vi "Create OPC UA Name.vi"(7 "Parent Type":T1, 11 "SV":string) -> (3 "Path":string, 4 "Folder":string, 5 "Name":string)   [LabVIEW 2016]
doc: "Generates an OPC UA name and position for the shared variable."
uses:
  Controls/Node Type.ctl
  <vilib>/OPCUA/NI OPC UA Utility.lvlib
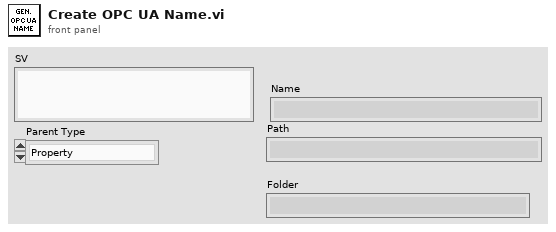
[diagram p1: front panel]
types:
  T1 = typedef "Node Type.ctl" = enum16{"Property", "Item", "Folder"}
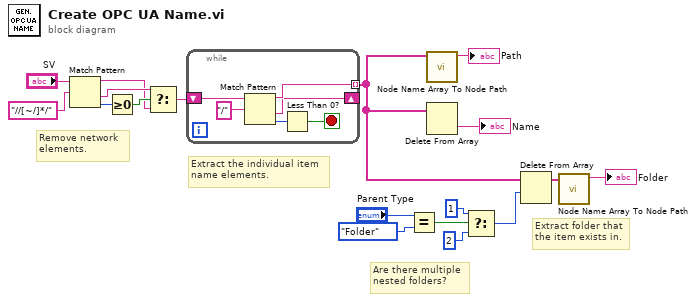
[diagram p0: block diagram]
diagram:
  # "Remove network\nelements."
  # "Extract the individual item\nname elements."
  # "Extract folder that\nthe item exists in."
  # "Are there multiple\nnested folders?"
  n1 = Match Pattern(string="SV", regular expression="//[~/]*/") -> (before substring=w14:string, after substring=w15:string, offset past match=w17:i32)  [unwired: 1 in, 1 out]
  n2 = Greater Or Equal To 0?(x=w17) -> (x >= 0?=w16:bool)
  n3 = Select(t=w15, s=w16, f=w14) -> (s? t:f=w10:string)
  n4 = while {
    shift-right: [w19] -> _
    shift-left: w10 -> [w24]
    tunnel: [w20] -> w8 mode=indexing
    stop <- w21 stop-if-true
    n5 = Match Pattern(string=w24, regular expression="/" ("regular expression (\"\")")) -> (before substring=w20:string, after substring=w19:string, offset past match=w22:i32)  [unwired: 1 in, 1 out]
    n6 = Less Than 0?(x=w22) -> (x < 0?=w21:bool)
  }
  n7 = Equal?(x="Parent Type", y=Node_Type."Folder") -> (x = y?=w4:bool)
  n8 = call <vilib>:"Node Name Array To Node Path.vi"("node names"=w8) -> ("node path"=→"Path":string)  [unwired: 9 in, 1 out]
  n9 = Delete From Array(array=w8) -> (deleted portion=→"Name":string)  [unwired: 2 in, 1 out]
  n10 = Select(t=1 ("length"), s=w4, f=2 ("length")) -> (s? t:f=w1:i32)
  n11 = Delete From Array(array=w8, length=w1) -> (array with subset deleted=w5:string[])  [unwired: 1 in, 1 out]
  n12 = call <vilib>:"Node Name Array To Node Path.vi"("node names"=w5) -> ("node path"=→"Folder":string)  [unwired: 9 in, 1 out]
